vi "Get_Sub_Collection.vi"(8 "error in (no error)":errorcluster caption="entrée d'erreur (pas d'erreur)", 11 "Firebase Benches en entrée":refnum<class "Firebase Packaging.lvclass">) -> (0 "error out":errorcluster caption="sortie d'erreur", 3 "Firebase Benches en sortie":refnum<class "Firebase Packaging.lvclass">)   [LabVIEW 2020, in "Library Instrument & Equipement.lvlib" / "Library FireBase.lvlib" / "Firebase Packaging.lvclass"]
doc: "Return the documents present in the test collection for each DATA read with Get_Data\nPlease initialise the following values\n - Name BDD\n - Document of test sequence\n - API Key\n - Nb To Read"
uses:
  Firebase Packaging.lvclass
  C:/Users/ngarcin/OneDrive - Altyor/Standard TB/Class/Firebase/Source/Firebase Driver/Firebase Driver.lvclass
  Firebase Packaging.lvclass/Firebase Packaging.ctl
  JSON API/JSON Value/JSON Value.lvclass
  JSON API/JSON Value/Set from JSON string.vi
  Firebase Altyor/Firebase Altyor.lvclass
  JSON API/Variant JSON/Variant JSON.lvlib
  JSON API/Get Polymorphic/JSON GetSet.lvlib
  Firebase Driver/Firebase Driver.lvclass
panel:
  out "documents":T1(array[cluster])
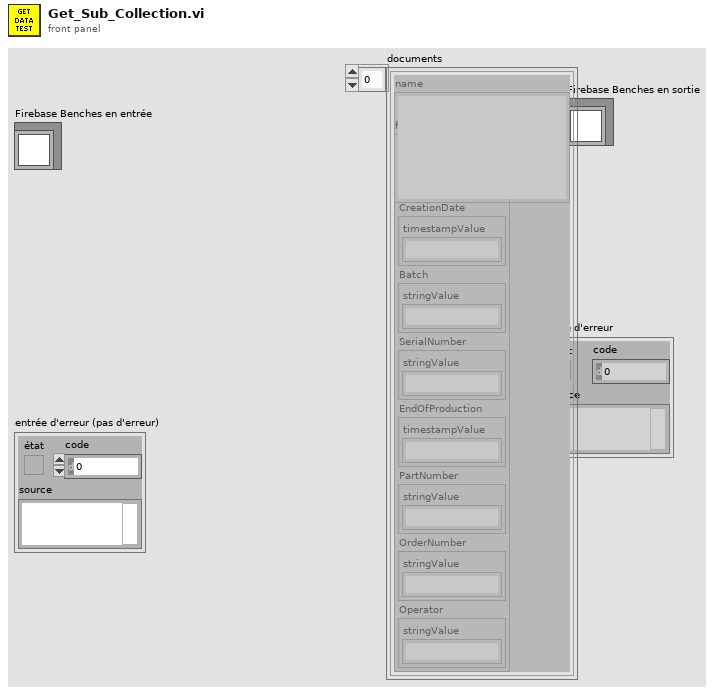
[diagram p1: front panel]
types:
  T1 = cluster{"name":string, "fields":cluster{"Result":cluster{"booleanValue":bool}, "CreationDate":cluster{"timestampValue":string}, "Batch":cluster{"stringValue":string}, "SerialNumber":cluster{"stringValue":string}, "EndOfProduction":cluster{"timestampValue":string}, "PartNumber":cluster{"stringValue":string}, "OrderNumber":cluster{"stringValue":string}, "Operator":cluster{"stringValue":string}}}[]
  T2 = cluster{"documents":cluster{"name":string, "fields":cluster{"Result":cluster{"booleanValue":bool}, "CreationDate":cluster{"timestampValue":string}, "Batch":cluster{"stringValue":string}, "SerialNumber":cluster{"stringValue":string}, "EndOfProduction":cluster{"timestampValue":string}, "PartNumber":cluster{"stringValue":string}, "OrderNumber":cluster{"stringValue":string}, "Operator":cluster{"stringValue":string}}}[]}
  T3 = cluster{"name":string, "fields":cluster{"SN_Produit":cluster{"stringValue":string}, "Product_Name":cluster{"stringValue":string}}}[][]
  T4 = cluster{"name":string, "fields":cluster{"SN_Produit":cluster{"stringValue":string}, "Product_Name":cluster{"stringValue":string}}}[]
  T5 = cluster{"documents":cluster{"name":string, "fields":cluster{"SN_Produit":cluster{"stringValue":string}, "Product_Name":cluster{"stringValue":string}}}[], "nextPageToken":string}
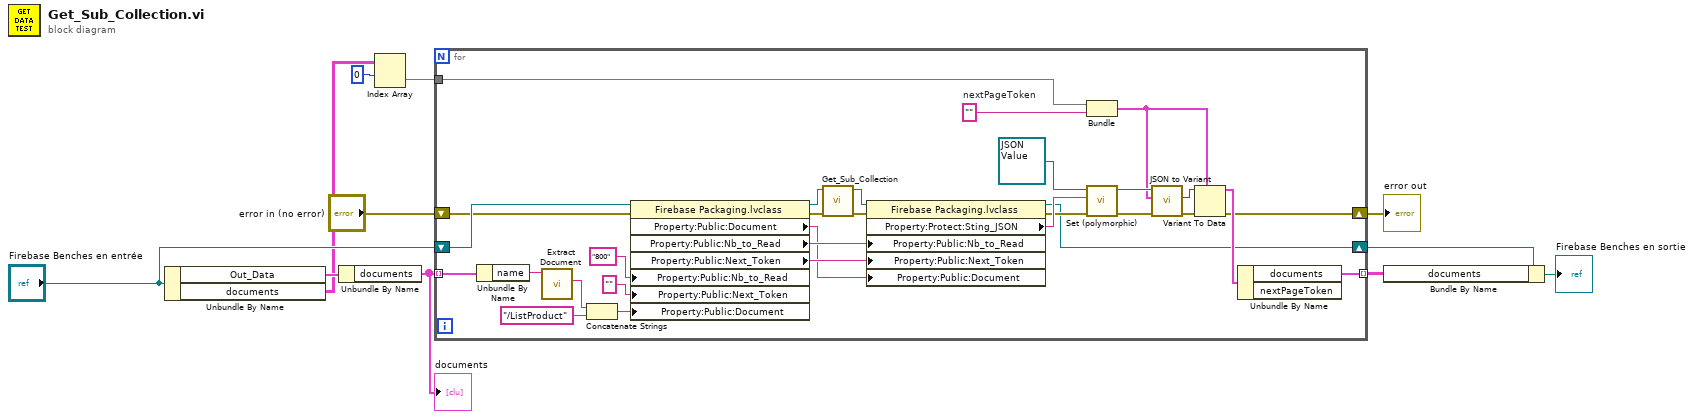
[diagram p0: block diagram]
diagram:
  n1 = Unbundle By Name("Firebase Benches en entrée") -> ("Out_Data"=w11:T2, "documents"=w4:T3)
  n2 = Unbundle By Name(w11) -> ("documents"=w10:T1)
  "documents" <- w10
  n3 = Index Array(array=w4, index (row)=0 ("indice (ligne)")) -> (element=w3:T4)  [unwired: 1 in]
  n4 = for {
    tunnel: [w16] -> w6 mode=indexing
    shift-right: [w13] -> w1
    shift-left: "Firebase Benches en entrée" -> [w34]
    shift-right: [w14] -> w9
    shift-left: "error in (no error)" -> [w33]
    tunnel: w10 -> [w32] mode=indexing
    tunnel: w3 -> [w19]
    w36 = ""  # nextPageToken
    n5 = Unbundle By Name(w32) -> ("name"=w31:string)
    n6 = call "Extract Document.vi"("Name"=w31) -> ("Source"=w30:string)  [unwired: 9 in, 1 out]
    n7 = Concatenate Strings(w30, "/ListProduct" ("chaîne")) -> (w28:string)
    n8 = property class="Firebase Packaging.lvclass"(reference=w34, error in=w33, "Property:Public:Nb_to_Read"="800" ("Nb_to_Read"), "Property:Public:Next_Token"="" ("Next_Token"), "Property:Public:Document"=w28) -> (reference out=w20:refnum<class "Firebase Packaging.lvclass">, error out=w23:errorcluster, "Property:Public:Document"=w12:string, "Property:Public:Nb_to_Read"=w27:string, "Property:Public:Next_Token"=w25:string)
    n9 = call-parent "Get_Sub_Collection.vi"("error in (no error)"=w23, "Firebase Altyor en entrée"=w20) -> ("error out"=w22:errorcluster, "Firebase Altyor en sortie"=w21:refnum<class "Firebase Packaging.lvclass">)  [unwired: 8 in]
    n10 = property class="Firebase Packaging.lvclass"(reference=w21, error in=w22, "Property:Public:Nb_to_Read"=w27, "Property:Public:Next_Token"=w25, "Property:Public:Document"=w12) -> (reference out=w13:refnum<class "Firebase Packaging.lvclass">, error out=w18:errorcluster, "Property:Protect:Sting_JSON"=w38:string)
    n11 = Bundle("documents"=w19, "nextPageToken"=w36) -> (w35:T5)  [unwired: 1 in]
    n12 = call-poly "Set (polymorphic).vi"("error in (no error)"=w18, "JSON stream"=w38, "JSON Value in"=refnum<class "JSON Value.lvclass"> refnum) -> ("error out"=w39:errorcluster, "JSON Value out"=w41:refnum<class "JSON Value.lvclass">)  [unwired: 6 in, 1 out]
    n13 = call "JSON to Variant.vi"("error in (no error)"=w39, "Variant (Data Type)"=w35, "JSON Value"=w41) -> ("error out"=w40:errorcluster, "Variant out"=w15:variant)  [unwired: 7 in]
    n14 = Variant To Data(error in=w40, type=w35, Variant=w15) -> (data=w37:T5, error out=w14:errorcluster)
    n15 = Unbundle By Name(w37) -> ("documents"=w16:T4)  [unwired: 1 out]
  }
  "error out" <- w9
  n16 = Bundle By Name(cluster=w1, "documents"=w6) -> (→"Firebase Benches en sortie":refnum<class "Firebase Packaging.lvclass">)
